vi "Set CPU Calculation State.vi"(8 "error in (no error)":errorcluster, 10 "Continuous":bool, 11 "Application Manager in":refnum<class "Application Manager.lvclass">) -> (0 "error out":errorcluster, 3 "Application Manager out":refnum<class "Application Manager.lvclass">)   [LabVIEW 2020, in "Application Manager.lvlib" / "Application Manager.lvclass"]
uses:
  Application Manager.lvclass
  Application Manager.lvclass/Application Manager.ctl
  Calculation Worker/Calculation Worker Messages/Set Calculation State Msg/Set Calculation State Msg.lvclass/Set Calculation State Msg.ctl
  <vilib>/ActorFramework/Message Enqueuer/Message Enqueuer.lvclass/Message Enqueuer.ctl
  <vilib>/ActorFramework/Message Enqueuer/Enqueue.vi
  Calculation Worker/Calculation Worker Messages/Set Calculation State Msg/Set Calculation State Msg.lvclass
  C:/Program Files/National Instruments/LabVIEW 2026/vi.lib/ActorFramework/Message/Message.lvclass
  <vilib>/ActorFramework/Message Priority Queue/Priority Enqueue.vi
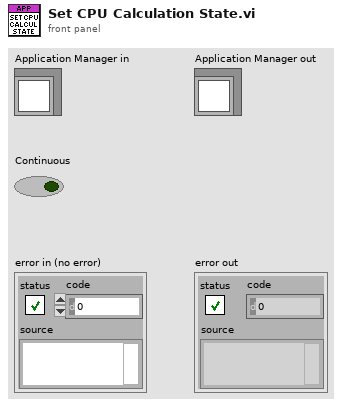
[diagram p1: front panel]
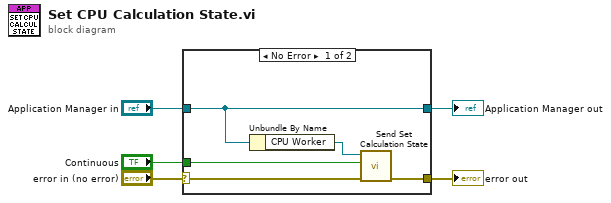
[diagram p0: block diagram]
diagram:
  n1 = case shown="No Error" "error in (no error)" {
    selector: "error in (no error)" -> [w8 w12]
    tunnel: [w6 w12] -> w4
    tunnel: [w9 w11] -> w2
    tunnel: "Application Manager in" -> [w9 w11]
    tunnel: "Continuous" -> [w7 _]
    frame No Error {
      n2 = Unbundle By Name(w9) -> ("CPU Worker"=w10:refnum<class "Message Enqueuer.lvclass">)
      n3 = call "Send Set Calculation State.vi"("error in (no error)"=w8, "Continuous"=w7, "Message Enqueuer"=w10) -> ("error out"=w6:errorcluster)  [unwired: 7 in, 1 out]
    }
    frame Error {
    }
  }
  "error out" <- w4
  "Application Manager out" <- w2
